vi "CalculaModulo.vi"(11 "Vetor de entrada":dbl[](array[numeric]) format="%#_13g") -> (3 "módulo":dbl format="%#_13g")   [LabVIEW 2018]
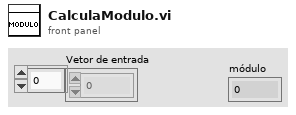
[diagram p1: front panel]
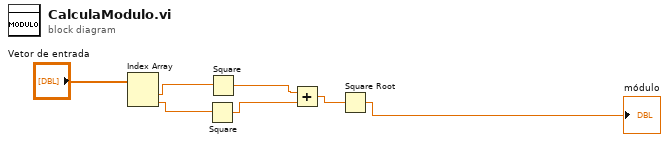
[diagram p0: block diagram]
diagram:
  n1 = Index Array(array="Vetor de entrada") -> (element #1=w6:dbl, element #2=w5:dbl)  [unwired: 2 in]
  n2 = Square(x=w5) -> (x^2=w3:dbl)
  n3 = Square(x=w6) -> (x^2=w4:dbl)
  n4 = Add(x=w4, y=w3) -> (x+y=w2:dbl)
  n5 = Square Root(x=w2) -> (sqrt(x)=→"módulo":dbl)
